vi "Taller 1 punto 1.vi"() -> ()   [LabVIEW 2017]
panel:
  in  "RATA DE T (°C/Seg)":dbl(knob) scale=1.0..10.0
  in  "SELECTOR":bool
  out "Sensor de temperatura °C":dbl(slide) scale=0.0..100.0
  # "TALLER 1, PUNTO 1\nLUZ ANDREA JARAMILLO CASTILLO"
  # "INCREMENTAR"
  # "DECREMENTAR"
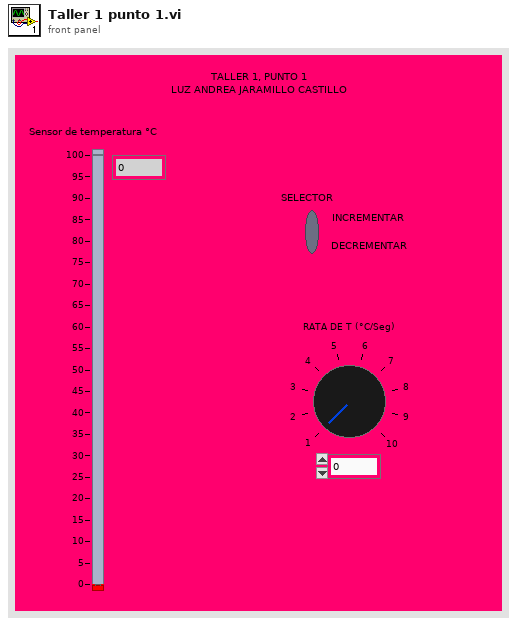
[diagram p1: front panel]
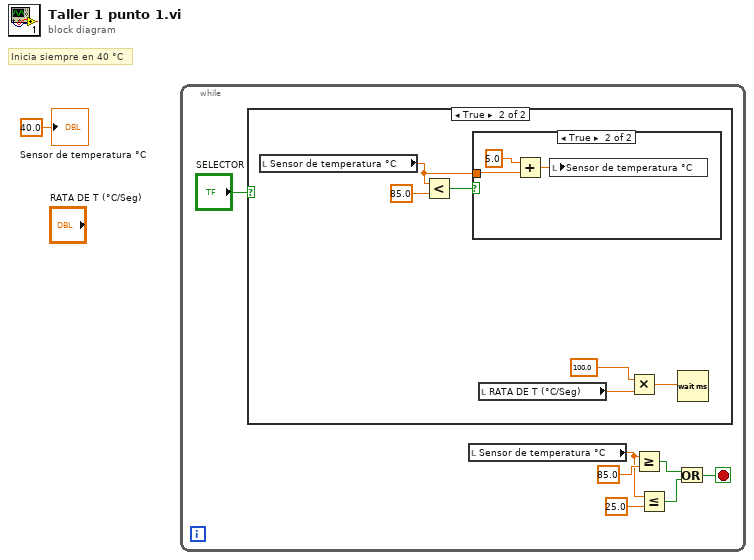
[diagram p0: block diagram]
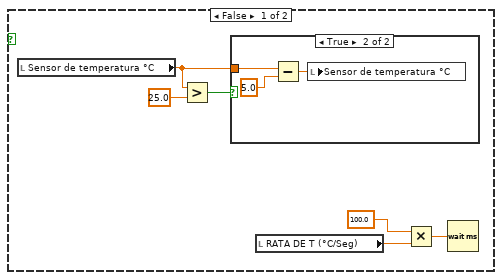
[diagram p2: hidden frame]
diagram:
  # "Inicia siempre en 40 °C"
  n1 = while {
    stop <- w2 stop-if-true
    n2 = case shown="True" "SELECTOR" {
      frame False {
        n3 = local read "Sensor de temperatura °C"() -> (w13:dbl)
        n4 = Greater?(x=w13, y=25.0) -> (0:w14:bool)
        n5 = case shown="True" w14 {
          tunnel: w13 -> [_ w16]
          frame False {
          }
          frame True {
            n6 = Subtract(x=w16, y=5.0 ("x")) -> (x-y=w17:dbl)
            n7 = local write "Sensor de temperatura °C"(w17) -> ()
          }
        }
        n8 = local read "RATA DE T (°C/Seg)"() -> (w11:dbl)
        n9 = Multiply(x=100.0, y=w11) -> (x*y=w9:dbl)
        n10 = Wait (ms)(milliseconds to wait=w9) -> ()  [unwired: 1 out]
      }
      frame True {
        n11 = local read "Sensor de temperatura °C"() -> (w21:dbl)
        n12 = Less?(x=w21, y=85.0) -> (x < y?=w22:bool)
        n13 = case shown="True" w22 {
          tunnel: w21 -> [_ w24]
          frame False {
          }
          frame True {
            n14 = Add(x=5.0, y=w24) -> (x+y=w26:dbl)
            n15 = local write "Sensor de temperatura °C"(w26) -> ()
          }
        }
        n16 = local read "RATA DE T (°C/Seg)"() -> (w20:dbl)
        n17 = Multiply(x=100.0, y=w20) -> (x*y=w18:dbl)
        n18 = Wait (ms)(milliseconds to wait=w18) -> ()  [unwired: 1 out]
      }
    }
    n19 = local read "Sensor de temperatura °C"() -> (w4:dbl)
    n20 = Greater Or Equal?(x=w4, y=85.0) -> (x >= y?=w6:bool)
    n21 = Less Or Equal?(x=w4, y=25.0) -> (x <= y?=w5:bool)
    n22 = Or(x=w6, y=w5) -> (x .or. y?=w2:bool)
  }
  "Sensor de temperatura °C" <- 40.0 ("Sensor de temperatura °C")
